vi "Raw Channel 2 proper channel.vi"(11 "channel in":u8) -> (0 "PPS?":bool, 3 "channel out":u8)   [LabVIEW 2016, in "HPTDC Driver Library.lvlib"]
uses:
  HPTDC Driver Library.lvlib
panel:
  # "Maps raw TDC channel IDs to scintillator channel IDs"
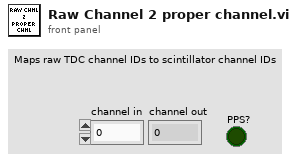
[diagram p1: front panel]
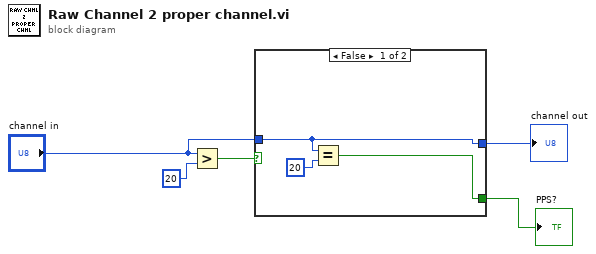
[diagram p0: block diagram]
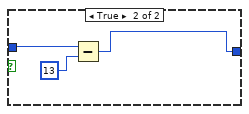
[diagram p2: hidden frame]
diagram:
  n1 = Greater?(x="channel in", y=u8 20) -> (0:w4:bool)
  n2 = case shown="False" w4 {
    tunnel: "channel in" -> [w8 w11]
    tunnel: [w8 w9] -> w2
    tunnel: [w6 _] -> w1
    frame False {
      n3 = Equal?(x=w8, y=20) -> (x = y?=w6:bool)
    }
    frame True {
      n4 = Subtract(x=w11, y=u8 13) -> (x-y=w9:u8)
    }
  }
  "channel out" <- w2
  "PPS?" <- w1
